vi "mdata.ini Write.vi"(0 "结果":string, 5 "data":string, 7 "sn":string, 9 "data_info":string, 11 "错误输入（无错误）":errorcluster) -> (15 "错误输出":errorcluster)   [LabVIEW 2019]
uses:
  <vilib>/Utility/config.llb/Write Key (String).vi
  <vilib>/Utility/config.llb/NI_LVConfig.lvlib
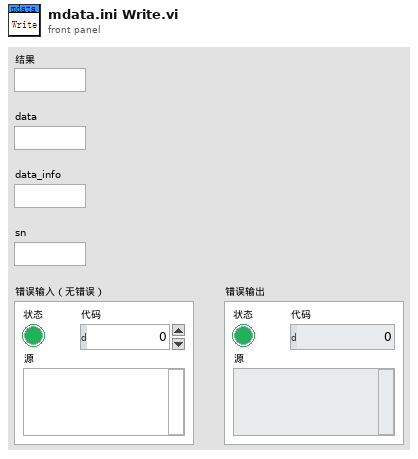
[diagram p1: front panel]
types:
  T1 = typedef "NI_LVConfig.lvlib/Config Data RefNum.ctl" = refnum<k1>
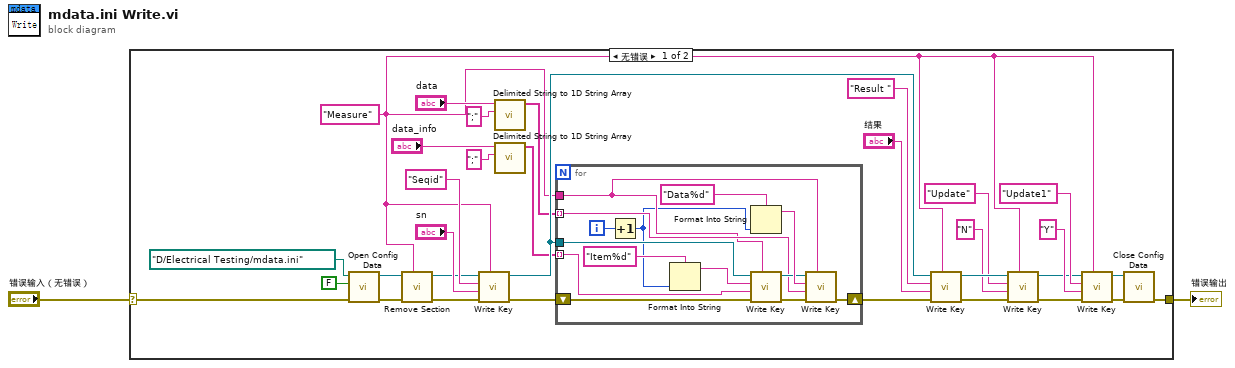
[diagram p0: block diagram]
diagram:
  n1 = case shown="无错误" "错误输入（无错误）" {
    selector: "错误输入（无错误）" -> [w8 w49]
    tunnel: [w9 w49] -> w2
    frame No Error {
      w3 = "Measure"
      n2 = call <vilib>:"Open Config Data.vi"("error in (no error)"=w8, "create file if necessary (T)"=FALSE, "configuration file path"=path "D:/Electrical Testing/mdata.ini") -> ("error out"=w34:errorcluster, "refnum"=w6:T1)  [unwired: 6 in, 1 out]
      n3 = call <vilib>:"Remove Section.vi"("section"=w3, "error in (no error)"=w34, "refnum"=w6) -> ("error out"=w4:errorcluster, "refnum out"=w5:T1)  [unwired: 6 in, 1 out]
      n4 = call-poly <vilib>:"Write Key.vi"("section"=w3, "error in (no error)"=w4, "value"="sn", "key"="Seqid", "refnum"=w5) -> ("error out"=w30:errorcluster, "refnum out"=w29:T1)  [unwired: 4 in, 1 out]
      n5 = call <vilib>:"Delimited String to 1D String Array.vi"("delimiter"=";", "delimited string"="data") -> ("string array"=w24:string[])  [unwired: 9 in]
      n6 = call <vilib>:"Delimited String to 1D String Array.vi"("delimiter"=";", "delimited string"="data_info") -> ("string array"=w23:string[])  [unwired: 9 in]
      n7 = for {
        tunnel: w29 -> [w48]
        tunnel: w3 -> [w36]
        tunnel: w23 -> [w44] mode=indexing
        tunnel: w24 -> [w38] mode=indexing
        shift-right: [w37] -> w33
        shift-left: w30 -> [w47]
        i -> [w42]
        n8 = Increment(x=w42) -> (x+1=w35:i32)
        n9 = Format Into String(format string="Item%d" ("格式字符串"), w35) -> (resulting string=w45:string)  [unwired: 2 in, 1 out]
        n10 = Format Into String(format string="Data%d" ("格式字符串"), w35) -> (resulting string=w41:string)  [unwired: 2 in, 1 out]
        n11 = call-poly <vilib>:"Write Key.vi"("section"=w36, "error in (no error)"=w47, "value"=w44, "key"=w45, "refnum"=w48) -> ("error out"=w39:errorcluster, "refnum out"=w40:T1)  [unwired: 4 in, 1 out]
        n12 = call-poly <vilib>:"Write Key.vi"("section"=w36, "error in (no error)"=w39, "value"=w38, "key"=w41, "refnum"=w40) -> ("error out"=w37:errorcluster)  [unwired: 4 in, 2 out]
      }
      n13 = call-poly <vilib>:"Write Key.vi"("section"=w3, "error in (no error)"=w33, "value"="结果", "key"="Result ", "refnum"=w29) -> ("error out"=w27:errorcluster, "refnum out"=w28:T1)  [unwired: 4 in, 1 out]
      n14 = call-poly <vilib>:"Write Key.vi"("section"=w3, "error in (no error)"=w27, "value"="N" ("key"), "key"="Update", "refnum"=w28) -> ("error out"=w17:errorcluster, "refnum out"=w16:T1)  [unwired: 4 in, 1 out]
      n15 = call-poly <vilib>:"Write Key.vi"("section"=w3, "error in (no error)"=w17, "value"="Y" ("key"), "key"="Update1", "refnum"=w16) -> ("error out"=w14:errorcluster, "refnum out"=w15:T1)  [unwired: 4 in, 1 out]
      n16 = call <vilib>:"Close Config Data.vi"("error in (no error)"=w14, "refnum"=w15) -> ("error out"=w9:errorcluster)  [unwired: 8 in, 1 out]
    }
    frame Error {
    }
  }
  "错误输出" <- w2
